vi "CreateTriggerCountNode.vi"(7 "DOM Document":refnum<k20>, 8 "Error In":errorcluster, 10 "Infinite?":bool, 11 "Count":u32) -> (0 "Error Out":errorcluster, 3 "Trigger Count Node":refnum<k20>)   [LabVIEW 2012]
uses:
  libs/LV-Utilities/LV-Utilities.lvlib
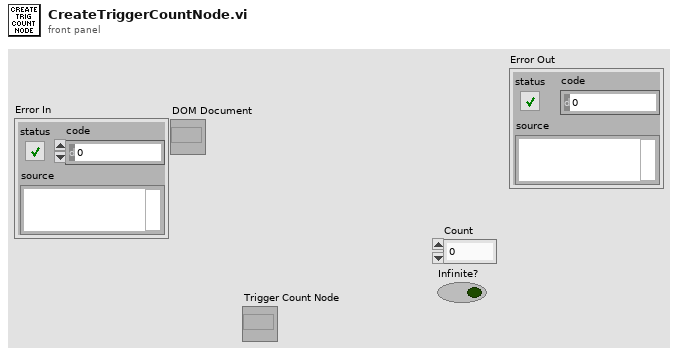
[diagram p1: front panel]
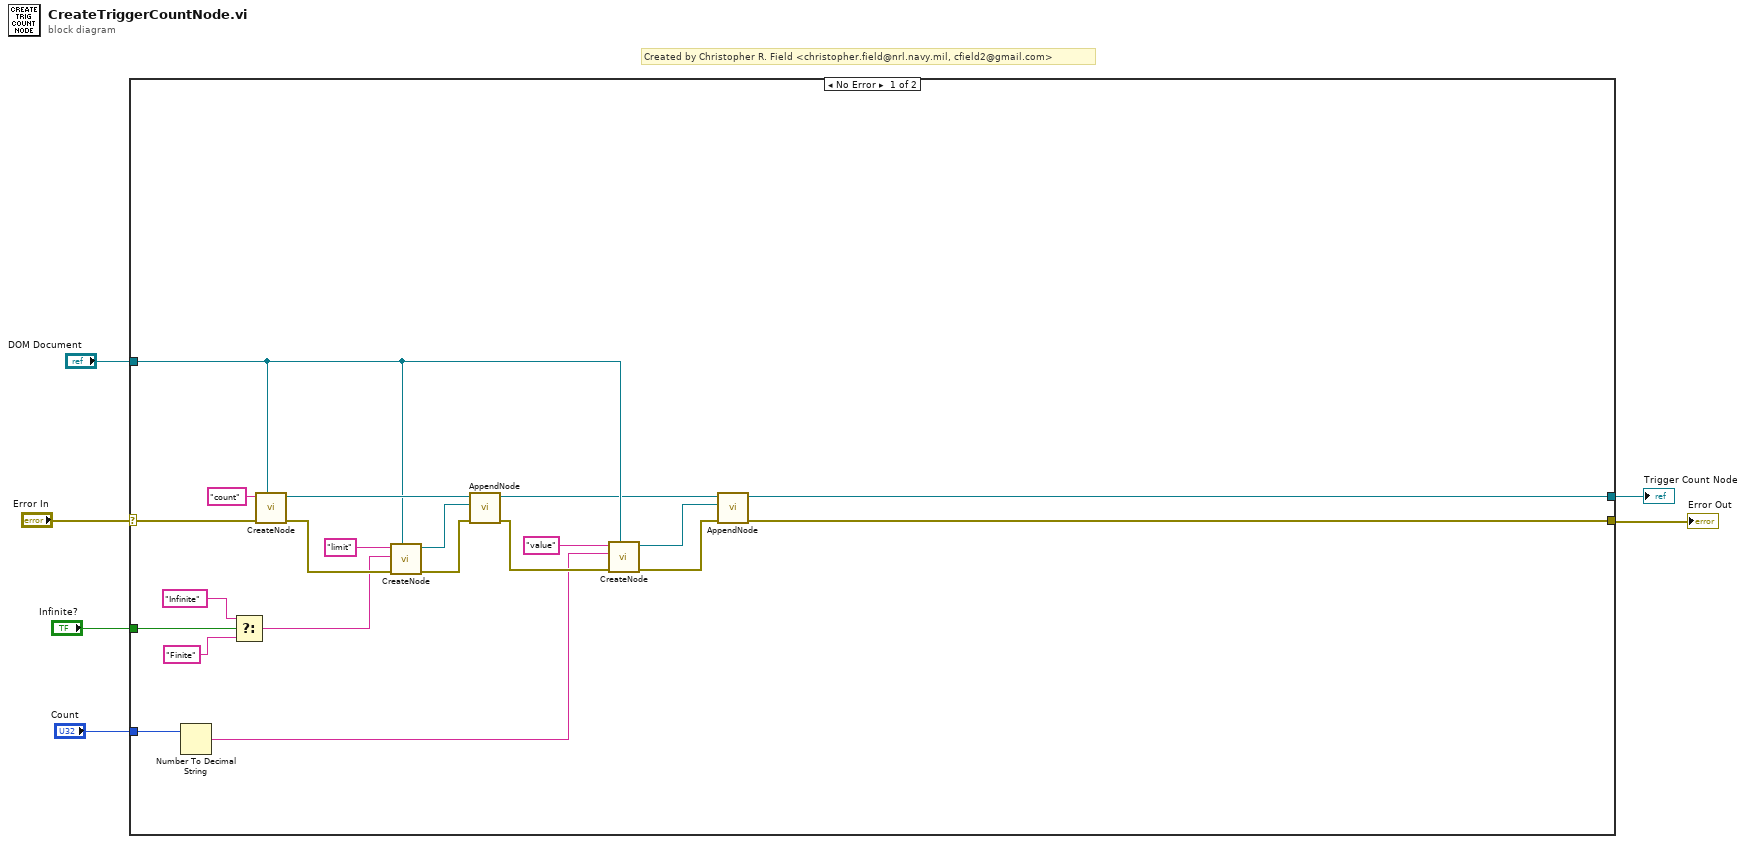
[diagram p0: block diagram]
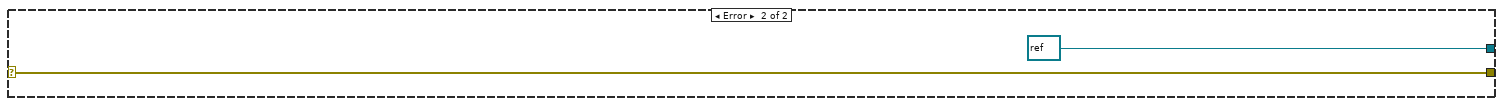
[diagram p2: hidden frame]
diagram:
  # "Created by Christopher R. Field <christopher.field@nrl.navy.mil, cfield2@gmail.com>"
  n1 = case shown="No Error" "Error In" {
    selector: "Error In" -> [w27 w29]
    tunnel: "DOM Document" -> [w13 _]
    tunnel: [w25 w29] -> w4
    tunnel: [w24 refnum<k20> refnum ("Wirings Node 2")] -> w3
    tunnel: "Count" -> [w20 _]
    tunnel: "Infinite?" -> [w19 _]
    frame No Error {
      n2 = Number To Decimal String(number=w20) -> (decimal integer string=w11:string)  [unwired: 1 in]
      n3 = Select(t="Infinite", s=w19, f="Finite") -> (s? t:f=w16:string)
      n4 = call "CreateNode.vi"("DOM Document"=w13, "Error In"=w27, "Tag Name"="count") -> ("Error out"=w22:errorcluster, "Node"=w23:refnum<k20>)  [unwired: 7 in]
      n5 = call "CreateNode.vi"("DOM Document"=w13, "Error In"=w22, "Text"=w16, "Tag Name"="limit") -> ("Error out"=w14:errorcluster, "Node"=w15:refnum<k20>)  [unwired: 6 in]
      n6 = call "AppendNode.vi"("Error In"=w14, "Child Node"=w15, "Parent Node In"=w23) -> ("Error Out"=w12:errorcluster, "Parent Node Out"=w9:refnum<k20>)  [unwired: 7 in]
      n7 = call "CreateNode.vi"("DOM Document"=w13, "Error In"=w12, "Text"=w11, "Tag Name"="value") -> ("Error out"=w8:errorcluster, "Node"=w7:refnum<k20>)  [unwired: 6 in]
      n8 = call "AppendNode.vi"("Error In"=w8, "Child Node"=w7, "Parent Node In"=w9) -> ("Error Out"=w25:errorcluster, "Parent Node Out"=w24:refnum<k20>)  [unwired: 7 in]
    }
    frame Error {
    }
  }
  "Trigger Count Node" <- w3
  "Error Out" <- w4
